vi "GetHighPrioritySensors.vi"   [LabVIEW 2020]
doc: "All high priority sensor reads and safety interlock calculations should be placed in this VI."
uses:
  <vilib>/Rock Robotics/WPI/DriverStation/WPI_DriverStationRobotMode2.ctl
  sensordata.vi
  robotoutputs.vi
  driverdata.vi
  refnumbers.vi
  GRNF_AI.vi
  GRNF_CTREMotor.vi
  <vilib>/Rock Robotics/WPI/ThirdParty/Phoenix-LabVIEW/Motor Controller/Get/CTRE_Phoenix_MotorController_GetSelectedSensorData.vi
  <vilib>/Rock Robotics/WPI/ThirdParty/Phoenix-LabVIEW/Motor Controller/Get/CTRE_Phoenix_MotorController_GetLimitSwitchStates.vi
  robotconstants.vi
types:
  T1 = typedef "WPI_DriverStationRobotMode2.ctl" = enum16{"Autonomous Disabled", "Autonomous Enabled", "Teleop Disabled", "Teleop Enabled", "Disconnected", "Finish", "Test Disabled", "Test Enabled", "Emergency Stopped"}
  T2 = enum16{"Low Gear", "High Gear", "Transiting", "Unknown", "Force Low Gear"}
  T3 = typedef "WPI_AnalogChannelDevRef.ctl" = cluster{"DevStatus":errorcluster, "Analog Channel":T4}
  T4 = typedef "FPGA_AIChannel.ctl" = enum8{"AI 0", "AI 1", "AI 2", "AI 3", "AI MXP 0", "AI MXP 1", "AI MXP 2", "AI MXP 3", "Invalid"}
  T5 = typedef "WPI_MotorControlDeviceRef.ctl" = cluster{"DeviceStatus":errorcluster, "Type":T6, "PWM":cluster{"PWM Channel":T7, "DeadBand":T8}, "CAN":cluster{"Device Number":u8, "SetOutput VI Ref":variant, "GetOutput VI Ref":variant, "Enable VI Ref":variant, "Disable VI Ref":variant, "Data":variant}, "Invert":bool, "DIO PWM":cluster{"PWM \"Enable\" Channel":T7, "DIOChannel":T9, "PWM Rate":dbl}}
  T6 = typedef "WPI_MotorControlType.ctl" = enum16{"PWM", "CAN", "DIO PWM"}
  T7 = typedef "FPGA_DIOPWMChannel.ctl" = enum8{"PWM 0", "PWM 1", "PWM 2", "PWM 3", "PWM 4", "PWM 5", "PWM 6", "PWM 7", "PWM 8", "PWM 9", "PWM MXP 0", "PWM MXP 1", "PWM MXP 2", "PWM MXP 3", "PWM MXP 4", "PWM MXP 5", "PWM MXP 6", "PWM MXP 7", "PWM MXP 8", "PWM MXP 9", "Invalid"}
  T8 = typedef "WPI_PWMDeadband.ctl" = cluster{"Name":string, "maxPositivePwm":i32, "minPositivePwm":i32, "centerPwm":i32, "maxNegativePwm":i32, "minNegativePwm":i32, "angularRange":u16}
  T9 = typedef "FPGA_DIOChannel.ctl" = enum8{"DIO 0", "DIO 1", "DIO 2", "DIO 3", "DIO 4", "DIO 5", "DIO 6", "DIO 7", "DIO 8", "DIO 9", "DIO MXP 0", "DIO MXP 1", "DIO MXP 2", "DIO MXP 3", "DIO MXP 4", "DIO MXP 5", "DIO MXP 6", "DIO MXP 7", "DIO MXP 8", "DIO MXP 9", "DIO MXP 10", "DIO MXP 11", "DIO MXP 12", "DIO MXP 13", "DIO MXP 14", "DIO MXP 15", "SPI Port CS1", "SPI Port CS2", "SPI Port CS3", "SPI Port MISO", "SPI Port MOSI", "Invalid"}
  T10 = typedef "Color Sensor V3 DevRef.ctl" = cluster{"I2CDevRef":T11}
  T11 = typedef "WPI_I2CDevRef.ctl" = cluster{"DevStatus":errorcluster, "Device Address":u8, "Handle":i32, "I2C Bus":T12}
  T12 = typedef "i2c_bus.ctl" = enum16{"I2C On-Board", "I2C MXP", "Invalid"}
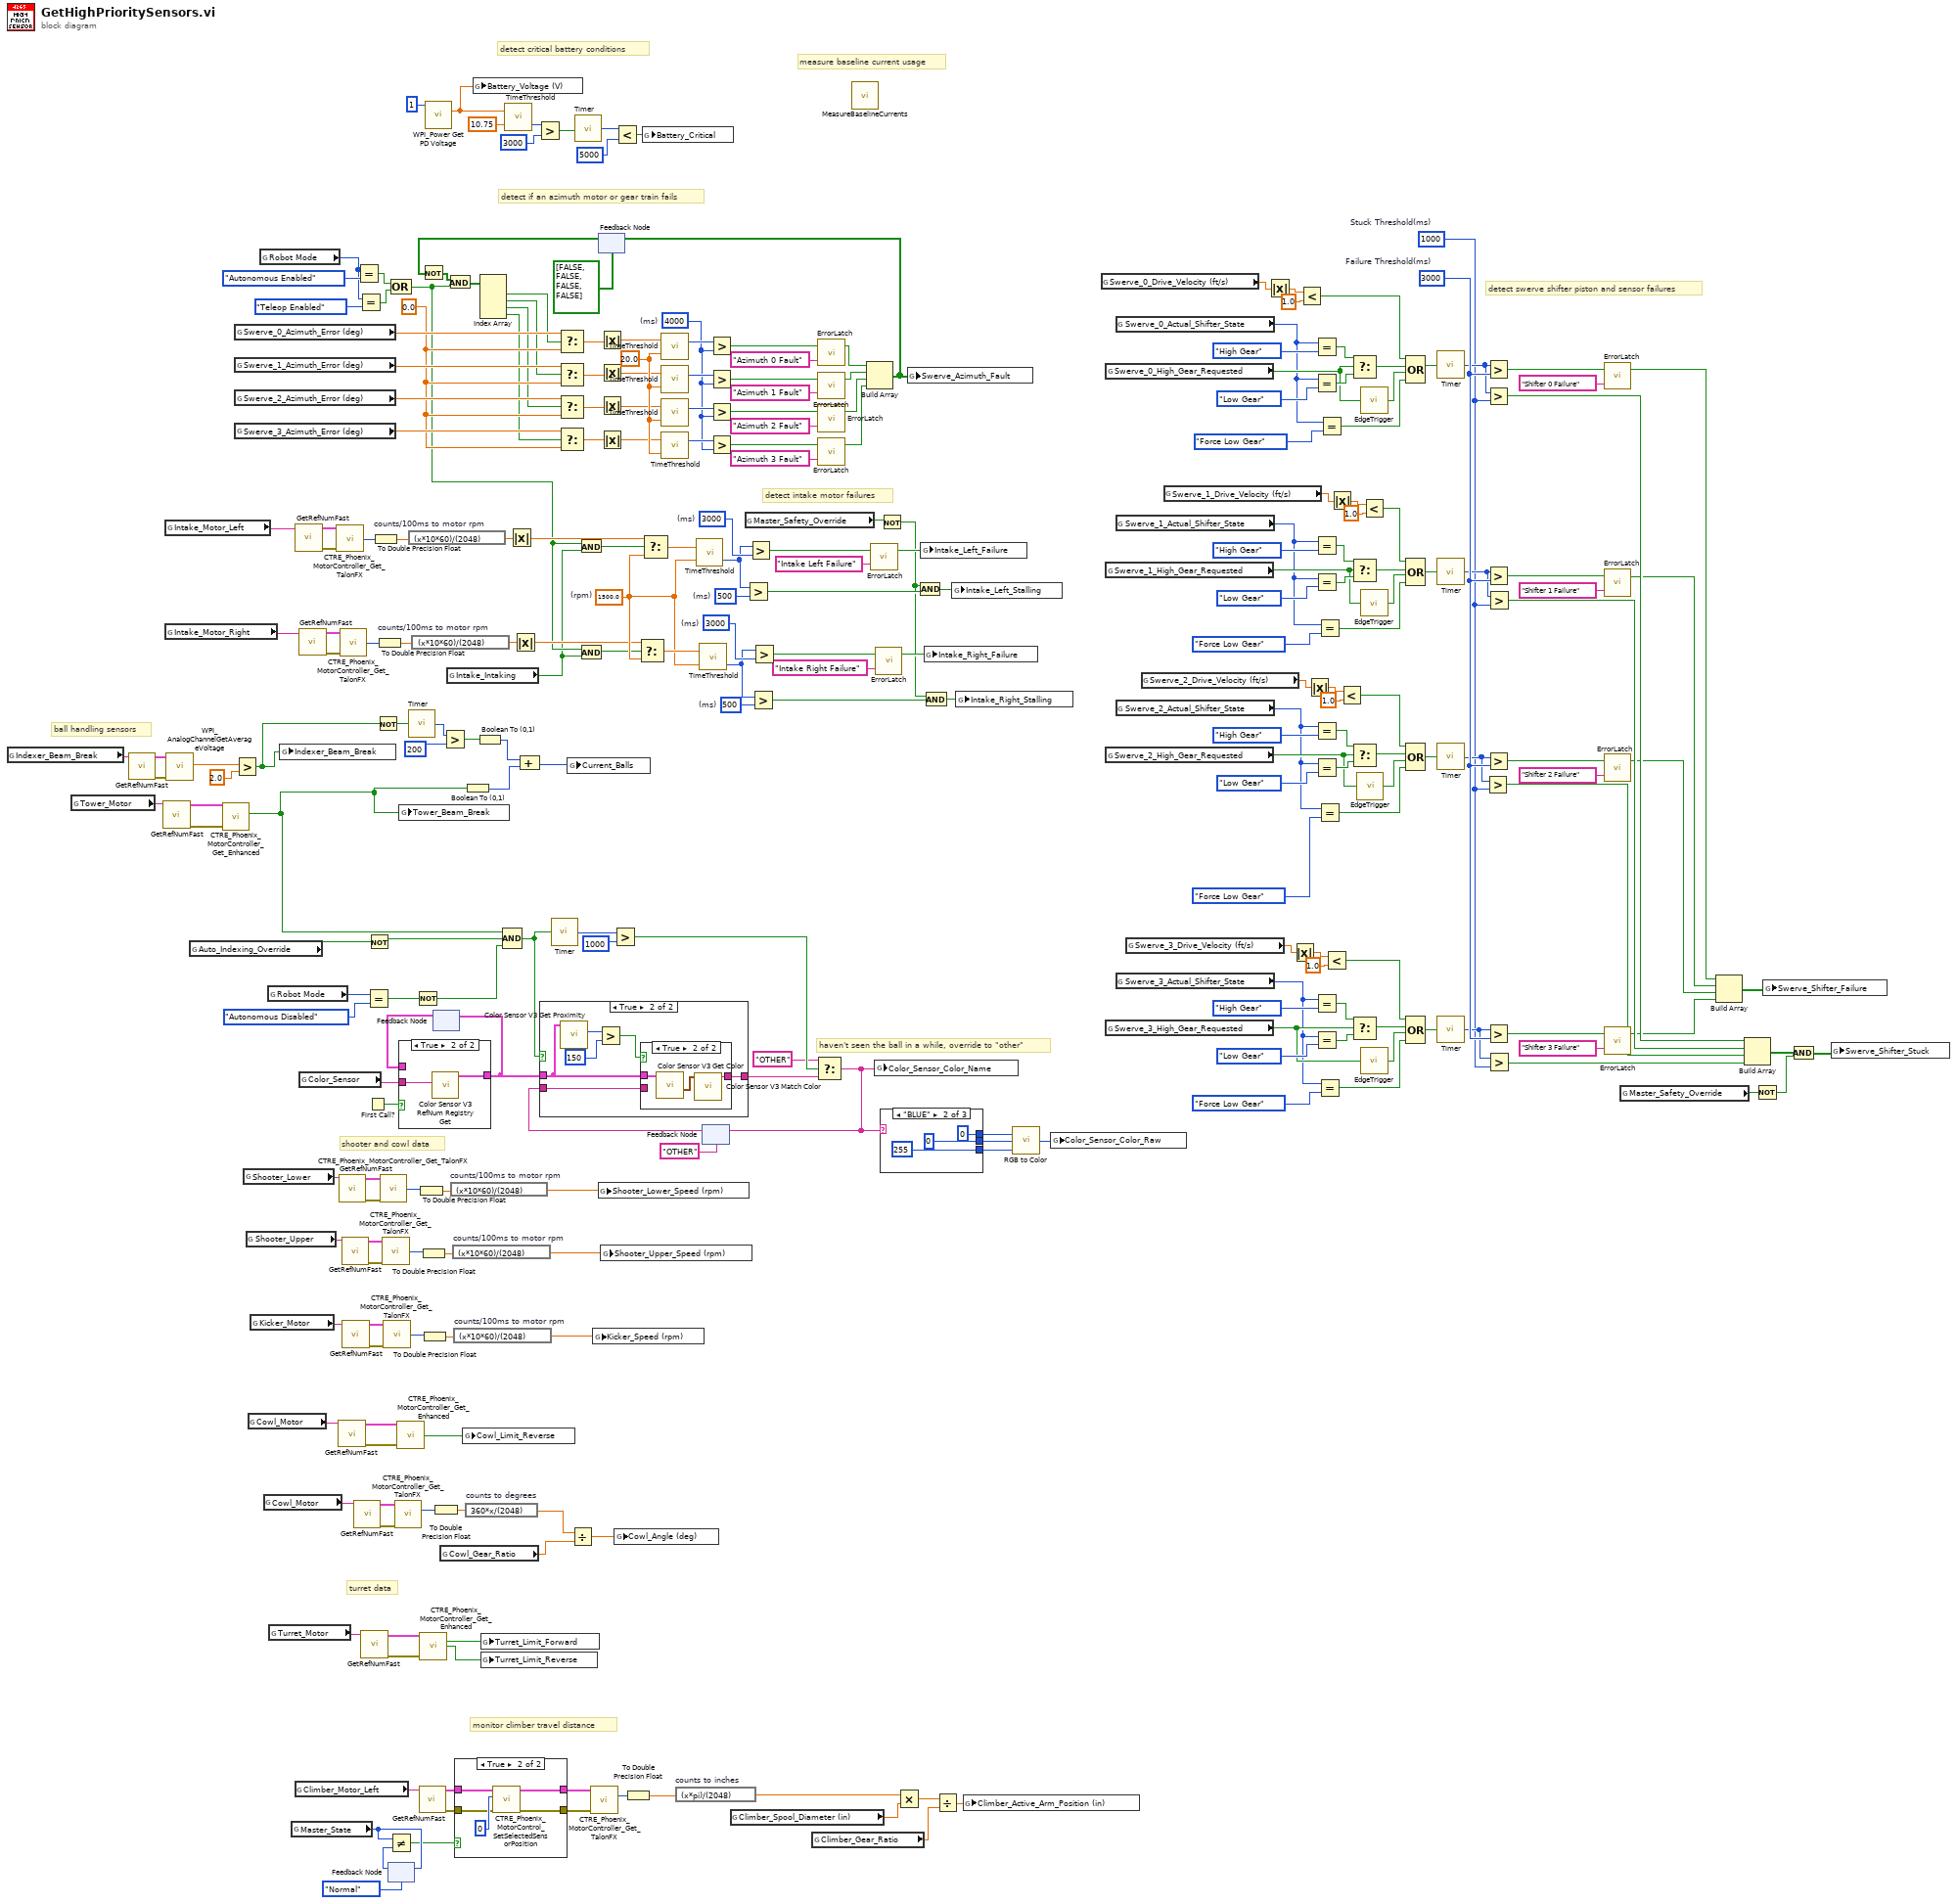
[diagram p0: block diagram]
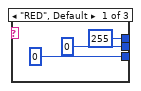
[diagram p5: hidden frame]
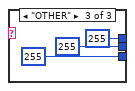
[diagram p6: hidden frame]
diagram:
  w22 = u32 500  # (ms)
  w24 = u32 500  # (ms)
  w129 = 1500.0  # (rpm)
  w136 = u32 3000  # (ms)
  w144 = u32 3000  # (ms)
  w198 = u32 1000  # Stuck Threshold(ms)
  w219 = u32 3000  # Failure Threshold(ms)
  w151 = 0.0
  w264 = u32 4000  # (ms)
  w263 = 20.0 ("Threshold")
  # "measure baseline current usage"
  # "monitor climber travel distance"
  # "haven't seen the ball in a while, override to \"other\""
  # "shooter and cowl data"
  # "turret data"
  # "detect intake motor failures"
  # "ball handling sensors"
  # "detect critical battery conditions"
  # "detect swerve shifter piston and sensor failures"
  # "detect if an azimuth motor or gear train fails"
  n1 = global read "refnumbers.vi" "Indexer_Beam_Break"() -> (w124:string)
  n2 = global read "refnumbers.vi" "Tower_Motor"() -> (w56:string)
  n3 = call-poly "GetRefNumFast.vi"("RefNum Name"=w124) -> ("Error"=w122:errorcluster, "Device Reference"=w123:T3)  [unwired: 5 in]
  n4 = call-poly "GetRefNumFast.vi"("RefNum Name"=w56) -> ("Error"=w54:errorcluster, "Device Reference"=w55:T5)  [unwired: 5 in]
  n5 = global read "refnumbers.vi" "Intake_Motor_Left"() -> (w149:string)
  n6 = global read "refnumbers.vi" "Intake_Motor_Right"() -> (w141:string)
  n7 = call <vilib>:"WPI_AnalogChannelGetAverageVoltage.vi"("error in (no error)"=w122, "AIDeviceRef"=w123) -> ("Voltage"=w150:dbl)  [unwired: 7 in, 2 out]
  n8 = global read "driverdata.vi" "Auto_Indexing_Override"() -> (w2:bool)
  n9 = call-poly <vilib>:"CTRE_Phoenix_MotorController_Get_Enhanced.vi"("PhoenixMotorControlDevRef"=w55, "error in"=w54) -> ("Forward Limit Closed?"=w3:bool)  [unwired: 10 in, 3 out]
  n10 = Greater?(x=w150, y=2.0) -> (0:w48:bool)
  n11 = global read "robotoutputs.vi" "Swerve_0_Azimuth_Error (deg)"() -> (w247:dbl)
  n12 = global read "robotoutputs.vi" "Swerve_1_Azimuth_Error (deg)"() -> (w246:dbl)
  n13 = global read "robotoutputs.vi" "Swerve_2_Azimuth_Error (deg)"() -> (w245:dbl)
  n14 = global read "robotoutputs.vi" "Swerve_3_Azimuth_Error (deg)"() -> (w244:dbl)
  n15 = global read "refnumbers.vi" "Shooter_Lower"() -> (w108:string)
  n16 = global read "refnumbers.vi" "Shooter_Upper"() -> (w102:string)
  n17 = global read "refnumbers.vi" "Cowl_Motor"() -> (w97:string)
  n18 = global read "refnumbers.vi" "Kicker_Motor"() -> (w7:string)
  n19 = global read "driverdata.vi" "Robot Mode"() -> (w256:T1)
  n20 = global read "refnumbers.vi" "Cowl_Motor"() -> (w94:string)
  n21 = global read "driverdata.vi" "Robot Mode"() -> (w79:T1)
  n22 = global read "refnumbers.vi" "Turret_Motor"() -> (w115:string)
  n23 = global write "sensordata.vi" "Indexer_Beam_Break"(w48) -> ()
  n24 = global read "robotoutputs.vi" "Master_State"() -> (w35:enum16{"Normal", "Climb"})
  n25 = global read "refnumbers.vi" "Climber_Motor_Left"() -> (w45:string)
  n26 = call-poly "GetRefNumFast.vi"("RefNum Name"=w149) -> ("Error"=w147:errorcluster, "Device Reference"=w148:T5)  [unwired: 5 in]
  n27 = call-poly "GetRefNumFast.vi"("RefNum Name"=w141) -> ("Error"=w139:errorcluster, "Device Reference"=w140:T5)  [unwired: 5 in]
  n28 = global read "refnumbers.vi" "Color_Sensor"() -> (w126:string)
  n29 = call-poly <vilib>:"CTRE_Phoenix_MotorController_Get_TalonFX.vi"("PhoenixMotorControlDevRef"=w148, "error in"=w147) -> ("Velocity (Raw Sensor Units per 100 ms)"=w146:i32)  [unwired: 10 in, 3 out]
  n30 = call-poly "GetRefNumFast.vi"("RefNum Name"=w97) -> ("Error"=w95:errorcluster, "Device Reference"=w96:T5)  [unwired: 5 in]
  n31 = call-poly "GetRefNumFast.vi"("RefNum Name"=w108) -> ("Error"=w106:errorcluster, "Device Reference"=w107:T5)  [unwired: 5 in]
  n32 = call-poly <vilib>:"CTRE_Phoenix_MotorController_Get_TalonFX.vi"("PhoenixMotorControlDevRef"=w140, "error in"=w139) -> ("Velocity (Raw Sensor Units per 100 ms)"=w138:i32)  [unwired: 10 in, 3 out]
  n33 = call-poly "GetRefNumFast.vi"("RefNum Name"=w102) -> ("Error"=w100:errorcluster, "Device Reference"=w101:T5)  [unwired: 5 in]
  n34 = call-poly "GetRefNumFast.vi"("RefNum Name"=w7) -> ("Error"=w5:errorcluster, "Device Reference"=w6:T5)  [unwired: 5 in]
  n35 = call-poly "GetRefNumFast.vi"("RefNum Name"=w94) -> ("Error"=w92:errorcluster, "Device Reference"=w93:T5)  [unwired: 5 in]
  n36 = Equal?(x=w256, y=WPI_DriverStationRobotMode2."Autonomous Enabled") -> (x = y?=w255:bool)
  n37 = Equal?(x=w256, y=WPI_DriverStationRobotMode2."Teleop Enabled") -> (x = y?=w254:bool)
  n38 = call-poly "GetRefNumFast.vi"("RefNum Name"=w115) -> ("Error"=w113:errorcluster, "Device Reference"=w114:T5)  [unwired: 5 in]
  n39 = Equal?(x=w79, y=WPI_DriverStationRobotMode2."Autonomous Disabled" ("Robot Mode")) -> (x = y?=w69:bool)
  n40 = First Call?() -> (First Call?: T/F=w127:bool)
  n41 = Not(x=w2) -> (.not. x?=w1:bool)
  n42 = To Double Precision Float(number=w146) -> (double precision float=w145:dbl)
  n43 = Not(x=w48) -> (.not. x?=w46:bool)
  n44 = To Double Precision Float(number=w138) -> (double precision float=w137:dbl)
  n45 = call-poly <vilib>:"CTRE_Phoenix_MotorController_Get_TalonFX.vi"("PhoenixMotorControlDevRef"=w107, "error in"=w106) -> ("Velocity (Raw Sensor Units per 100 ms)"=w109:i32)  [unwired: 10 in, 3 out]
  n46 = call-poly <vilib>:"CTRE_Phoenix_MotorController_Get_TalonFX.vi"("PhoenixMotorControlDevRef"=w101, "error in"=w100) -> ("Velocity (Raw Sensor Units per 100 ms)"=w103:i32)  [unwired: 10 in, 3 out]
  n47 = call-poly <vilib>:"CTRE_Phoenix_MotorController_Get_TalonFX.vi"("PhoenixMotorControlDevRef"=w6, "error in"=w5) -> ("Velocity (Raw Sensor Units per 100 ms)"=w8:i32)  [unwired: 10 in, 3 out]
  n48 = feedback #1(enum16{"Normal", "Climb"}."Normal" ("Master_State")) -> (w36:enum16{"Normal", "Climb"})
  n49 = Not Equal?(x=w35, y=w36) -> (x != y?=w34:bool)
  n50 = feedback-in #1(w35) -> ()
  n51 = Compound Arithmetic op=OR(w255, w254) -> (w25:bool)
  n52 = call-poly <vilib>:"CTRE_Phoenix_MotorController_Get_TalonFX.vi"("PhoenixMotorControlDevRef"=w93, "error in"=w92) -> ("Position (Raw Sensor Units)"=w91:i32)  [unwired: 10 in, 3 out]
  n53 = call-poly <vilib>:"CTRE_Phoenix_MotorController_Get_Enhanced.vi"("PhoenixMotorControlDevRef"=w96, "error in"=w95) -> ("Reverse Limit Closed?"=w98:bool)  [unwired: 10 in, 3 out]
  n54 = global write "sensordata.vi" "Tower_Beam_Break"(w3) -> ()
  n55 = expression code="(x*10*60)/(2048)" "counts/100ms to motor rpm"(w145) -> (w128:dbl)
  n56 = call "Timer.vi"("Reset Timer"=w46) -> ("Time (ms)"=w53:u32)
  n57 = expression code="(x*10*60)/(2048)" "counts/100ms to motor rpm"(w137) -> (w133:dbl)
  n58 = Not(x=w69) -> (.not. x?=w29:bool)
  n59 = To Double Precision Float(number=w109) -> (double precision float=w110:dbl)
  n60 = call-poly "GetRefNumFast.vi"("RefNum Name"=w45) -> ("Error"=w39:errorcluster, "Device Reference"=w40:T5)  [unwired: 5 in]
  n61 = call-poly <vilib>:"CTRE_Phoenix_MotorController_Get_Enhanced.vi"("PhoenixMotorControlDevRef"=w114, "error in"=w113) -> ("Forward Limit Closed?"=w112:bool, "Reverse Limit Closed?"=w111:bool)  [unwired: 10 in, 2 out]
  n62 = To Double Precision Float(number=w103) -> (double precision float=w104:dbl)
  n63 = To Double Precision Float(number=w8) -> (double precision float=w9:dbl)
  n64 = call <vilib>:"WPI_Power Get PD Voltage.vi"("Power Distribution Panel (def)"=u8 1) -> ("voltage (V)"=w153:dbl)  [unwired: 13 in, 1 out]
  n65 = feedback #2() -> (w125:T10)  [unwired: 1 in]
  n66 = case shown="True" w127 {
    tunnel: [w272 w273] -> w68
    tunnel: w125 -> [w272 _]
    tunnel: w126 -> [_ w274]
    frame False {
    }
    frame True {
      n67 = call <vilib>:"Color Sensor V3 RefNum Registry Get.vi"("refnum name"=w274) -> ("ColorSensorDevRef"=w273:T10)  [unwired: 9 in, 1 out]
    }
  }
  n68 = feedback-in #2(w68) -> ()
  n69 = To Double Precision Float(number=w91) -> (double precision float=w90:dbl)
  n70 = global read "robotconstants.vi" "Cowl_Gear_Ratio"() -> (w88:dbl)
  n71 = Greater?(x=w53, y=u32 200) -> (0:w52:bool)
  n72 = global read "robotoutputs.vi" "Intake_Intaking"() -> (w20:bool)
  n73 = expression code="(x*10*60)/(2048)" "counts/100ms to motor rpm"(w110) -> (w105:dbl)
  n74 = expression code="(x*10*60)/(2048)" "counts/100ms to motor rpm"(w104) -> (w99:dbl)
  n75 = expression code="(x*10*60)/(2048)" "counts/100ms to motor rpm"(w9) -> (w4:dbl)
  n76 = case shown="True" w34 {
    tunnel: w40 -> [w276 w280]
    tunnel: w39 -> [w275 w279]
    tunnel: [w276 w278] -> w37
    tunnel: [w275 w277] -> w38
    frame False {
    }
    frame True {
      n77 = call <vilib>:"CTRE_Phoenix_MotorControl_SetSelectedSensorPosition.vi"("error in (no error)"=w279, "New Sensor Position"=0, "PhoenixMotorControlDevRef"=w280) -> ("error out"=w277:errorcluster, "PhoenixMotorControlDevRef"=w278:T5)  [unwired: 7 in]
    }
  }
  n78 = global write "sensordata.vi" "Cowl_Limit_Reverse"(w98) -> ()
  n79 = Boolean To (0,1)(Boolean=w3) -> (0, 1=w50:i16)
  n80 = expression code="360*x/(2048)" "counts to degrees"(w90) -> (w89:dbl)
  n81 = global write "sensordata.vi" "Battery_Voltage (V)"(w153) -> ()
  n82 = Boolean To (0,1)(Boolean=w52) -> (0, 1=w51:i16)
  n83 = global write "sensordata.vi" "Turret_Limit_Forward"(w112) -> ()
  n84 = global write "sensordata.vi" "Turret_Limit_Reverse"(w111) -> ()
  n85 = Compound Arithmetic op=AND(w3, w1, w29) -> (w67:bool)
  n86 = call "TimeThreshold.vi"("Threshold"=10.75, "Current Value"=w153) -> ("Time Below Threshold (ms)"=w270:u32)  [unwired: 1 out]
  n87 = Absolute Value(x=w128) -> (abs(x)=w28:dbl)
  n88 = Absolute Value(x=w133) -> (abs(x)=w27:dbl)
  n89 = Compound Arithmetic op=ADD(w51, w50) -> (w49:i16)
  n90 = Greater?(x=w270, y=u32 3000) -> (0:w13:bool)
  n91 = call "Timer.vi"("Reset Timer"=w67) -> ("Time (ms)"=w86:u32)
  n92 = global write "sensordata.vi" "Current_Balls"(w49) -> ()
  n93 = Divide(x=w89, y=w88) -> (x/y=w87:dbl)
  n94 = call "Timer.vi"("Reset Timer"=w13) -> ("Time (ms)"=w12:u32)
  n95 = And(x=w25, y=w20) -> (x .and. y?=w130:bool)
  n96 = And(x=w25, y=w20) -> (x .and. y?=w26:bool)
  n97 = call-poly <vilib>:"CTRE_Phoenix_MotorController_Get_TalonFX.vi"("PhoenixMotorControlDevRef"=w37, "error in"=w38) -> ("Position (Raw Sensor Units)"=w43:i32)  [unwired: 10 in, 3 out]
  n98 = global write "sensordata.vi" "Kicker_Speed (rpm)"(w4) -> ()
  n99 = feedback #3(bool[] [FALSE, FALSE, FALSE, FALSE]) -> (w77:bool[])
  n100 = Not(x=w77) -> (.not. x?=w76:bool[])
  n101 = And(x=w76, y=w25) -> (x .and. y?=w75:bool[])
  n102 = Index Array(array=w75) -> (element #1=w71:bool, element #2=w72:bool, element #3=w73:bool, element #4=w74:bool)  [unwired: 4 in]
  n103 = Select(t=w247, s=w71, f=w151) -> (s? t:f=w243:dbl)
  n104 = Select(t=w246, s=w72, f=w151) -> (s? t:f=w242:dbl)
  n105 = Select(t=w245, s=w73, f=w151) -> (s? t:f=w241:dbl)
  n106 = Select(t=w244, s=w74, f=w151) -> (s? t:f=w240:dbl)
  n107 = global write "sensordata.vi" "Shooter_Lower_Speed (rpm)"(w105) -> ()
  n108 = Absolute Value(x=w243) -> (abs(x)=w262:dbl)
  n109 = Absolute Value(x=w242) -> (abs(x)=w261:dbl)
  n110 = Absolute Value(x=w241) -> (abs(x)=w260:dbl)
  n111 = Absolute Value(x=w240) -> (abs(x)=w259:dbl)
  n112 = global write "sensordata.vi" "Shooter_Upper_Speed (rpm)"(w99) -> ()
  n113 = Greater?(x=w86, y=u32 1000) -> (0:w84:bool)
  n114 = Less?(x=w12, y=u32 5000) -> (x < y?=w11:bool)
  n115 = global write "sensordata.vi" "Cowl_Angle (deg)"(w87) -> ()
  n116 = To Double Precision Float(number=w43) -> (double precision float=w44:dbl)
  n117 = Select(t=w27, s=w26, f=w129) -> (s? t:f=w131:dbl)
  n118 = global write "sensordata.vi" "Battery_Critical"(w11) -> ()
  n119 = Select(t=w28, s=w130, f=w129) -> (s? t:f=w132:dbl)
  n120 = call "TimeThreshold.vi"("Threshold"=w263, "Current Value"=w262) -> ("Time Above Threshold (ms)"=w268:u32)  [unwired: 1 out]
  n121 = call "TimeThreshold.vi"("Threshold"=w263, "Current Value"=w261) -> ("Time Above Threshold (ms)"=w267:u32)  [unwired: 1 out]
  n122 = call "TimeThreshold.vi"("Threshold"=w263, "Current Value"=w260) -> ("Time Above Threshold (ms)"=w266:u32)  [unwired: 1 out]
  n123 = call "TimeThreshold.vi"("Threshold"=w263, "Current Value"=w259) -> ("Time Above Threshold (ms)"=w265:u32)  [unwired: 1 out]
  n124 = expression code="(x*pi)/(2048)" "counts to inches"(w44) -> (w32:dbl)
  n125 = call "TimeThreshold.vi"("Threshold"=w129, "Current Value"=w132) -> ("Time Below Threshold (ms)"=w23:u32)  [unwired: 1 out]
  n126 = call "TimeThreshold.vi"("Threshold"=w129, "Current Value"=w131) -> ("Time Below Threshold (ms)"=w21:u32)  [unwired: 1 out]
  n127 = feedback #4("OTHER" ("Matched Color Name")) -> (w116:string)
  n128 = case shown="True" w67 {
    tunnel: w68 -> [_ w287]
    tunnel: [w282 w288] -> w81
    tunnel: w116 -> [w282 w286]
    frame False {
    }
    frame True {
      n129 = call <vilib>:"Color Sensor V3 Get Proximity.vi"("ColorSensorDevRef"=w287) -> ("Proximity"=w285:u16)  [unwired: 8 in, 2 out]
      n130 = Greater?(x=w285, y=u16 150) -> (0:w283:bool)
      n131 = case shown="True" w283 {
        tunnel: [w289 w291] -> w288
        tunnel: w287 -> [_ w290]
        tunnel: w286 -> [w289 _]
        frame False {
        }
        frame True {
          n132 = call <vilib>:"Color Sensor V3 Get Color.vi"("ColorSensorDevRef"=w290) -> ("Normalized Color"=w292:cluster{"R":dbl, "G":dbl, "B":dbl})  [unwired: 7 in, 3 out]
          n133 = call <vilib>:"Color Sensor V3 Match Color.vi"("Measured Color"=w292) -> ("Matched Color Name"=w291:string)  [unwired: 8 in, 2 out]
        }
      }
    }
  }
  n134 = Greater?(x=w268, y=w264) -> (0:w250:bool)
  n135 = Greater?(x=w267, y=w264) -> (0:w249:bool)
  n136 = Greater?(x=w266, y=w264) -> (0:w155:bool)
  n137 = Greater?(x=w265, y=w264) -> (0:w248:bool)
  n138 = global read "robotconstants.vi" "Climber_Spool_Diameter (in)"() -> (w30:dbl)
  n139 = global read "driverdata.vi" "Master_Safety_Override"() -> (w19:bool)
  n140 = Greater?(x=w23, y=w24) -> (0:w17:bool)
  n141 = Greater?(x=w23, y=w144) -> (0:w143:bool)
  n142 = Greater?(x=w21, y=w22) -> (0:w15:bool)
  n143 = Greater?(x=w21, y=w136) -> (0:w135:bool)
  n144 = global read "robotconstants.vi" "Climber_Gear_Ratio"() -> (w42:dbl)
  n145 = Select(t="OTHER" ("Matched Color Name"), s=w84, f=w81) -> (s? t:f=w82:string)
  n146 = feedback-in #4(w82) -> ()
  n147 = call "ErrorLatch.vi"("Error Message"="Azimuth 0 Fault", "Trigger"=w250) -> ("Latched"=w176:bool)  [unwired: 1 in]
  n148 = call "ErrorLatch.vi"("Error Message"="Azimuth 1 Fault", "Trigger"=w249) -> ("Latched"=w253:bool)  [unwired: 1 in]
  n149 = call "ErrorLatch.vi"("Error Message"="Azimuth 2 Fault", "Trigger"=w155) -> ("Latched"=w252:bool)  [unwired: 1 in]
  n150 = call "ErrorLatch.vi"("Error Message"="Azimuth 3 Fault", "Trigger"=w248) -> ("Latched"=w251:bool)  [unwired: 1 in]
  n151 = call "MeasureBaselineCurrents.vi"() -> ()  [unwired: 12 in]
  n152 = Build Array(w176, w253, w252, w251) -> (w78:bool[])
  n153 = feedback-in #3(w78) -> ()
  n154 = call "ErrorLatch.vi"("Error Message"="Intake Left Failure", "Trigger"=w143) -> ("Latched"=w142:bool)  [unwired: 1 in]
  n155 = global write "sensordata.vi" "Color_Sensor_Color_Name"(w82) -> ()
  n156 = call "ErrorLatch.vi"("Error Message"="Intake Right Failure", "Trigger"=w135) -> ("Latched"=w134:bool)  [unwired: 1 in]
  n157 = Not(x=w19) -> (.not. x?=w16:bool)
  n158 = case shown="\"BLUE\"" w82 {
    tunnel: [u8 255 ("R") u8 0 ("R") u8 255 ("R")] -> w120
    tunnel: [u8 0 ("R") u8 0 ("R") u8 255 ("R")] -> w119
    tunnel: [u8 0 ("R") u8 255 ("R") u8 255 ("R")] -> w118
    frame "RED", Default {
    }
    frame "BLUE" {
    }
    frame "OTHER" {
    }
  }
  n159 = Multiply(x=w32, y=w30) -> (x*y=w31:dbl)
  n160 = global write "sensordata.vi" "Swerve_Azimuth_Fault"(w78) -> ()
  n161 = And(x=w16, y=w17) -> (x .and. y?=w18:bool)
  n162 = global write "sensordata.vi" "Intake_Left_Failure"(w142) -> ()
  n163 = And(x=w16, y=w15) -> (x .and. y?=w14:bool)
  n164 = global write "sensordata.vi" "Intake_Right_Failure"(w134) -> ()
  n165 = Divide(x=w31, y=w42) -> (x/y=w41:dbl)
  n166 = global write "sensordata.vi" "Intake_Left_Stalling"(w18) -> ()
  n167 = global write "sensordata.vi" "Intake_Right_Stalling"(w14) -> ()
  n168 = global write "sensordata.vi" "Climber_Active_Arm_Position (in)"(w41) -> ()
  n169 = call <vilib>:"RGB to Color.vi"("B"=w118, "G"=w119, "R"=w120) -> ("Color"=w121:u32)
  n170 = global write "sensordata.vi" "Color_Sensor_Color_Raw"(w121) -> ()
  n171 = global read "sensordata.vi" "Swerve_0_Drive_Velocity (ft/s)"() -> (w193:dbl)
  n172 = global read "robotoutputs.vi" "Swerve_0_High_Gear_Requested"() -> (w218:bool)
  n173 = global read "robotoutputs.vi" "Swerve_1_High_Gear_Requested"() -> (w211:bool)
  n174 = global read "robotoutputs.vi" "Swerve_2_High_Gear_Requested"() -> (w208:bool)
  n175 = global read "robotoutputs.vi" "Swerve_3_High_Gear_Requested"() -> (w203:bool)
  n176 = global read "sensordata.vi" "Swerve_0_Actual_Shifter_State"() -> (w165:T2)
  n177 = global read "sensordata.vi" "Swerve_1_Actual_Shifter_State"() -> (w168:T2)
  n178 = global read "sensordata.vi" "Swerve_2_Actual_Shifter_State"() -> (w171:T2)
  n179 = global read "sensordata.vi" "Swerve_3_Actual_Shifter_State"() -> (w174:T2)
  n180 = global read "sensordata.vi" "Swerve_3_Drive_Velocity (ft/s)"() -> (w181:dbl)
  n181 = global read "sensordata.vi" "Swerve_2_Drive_Velocity (ft/s)"() -> (w185:dbl)
  n182 = global read "sensordata.vi" "Swerve_1_Drive_Velocity (ft/s)"() -> (w189:dbl)
  n183 = Absolute Value(x=w193) -> (abs(x)=w192:dbl)
  n184 = Absolute Value(x=w181) -> (abs(x)=w180:dbl)
  n185 = Less?(x=w192, y=1.0) -> (x < y?=w190:bool)
  n186 = Absolute Value(x=w185) -> (abs(x)=w184:dbl)
  n187 = Equal?(x=w165, y=T2."High Gear") -> (x = y?=w238:bool)
  n188 = Equal?(x=w165, y=T2."Low Gear") -> (x = y?=w236:bool)
  n189 = Equal?(x=w168, y=T2."High Gear") -> (x = y?=w233:bool)
  n190 = Equal?(x=w168, y=T2."Low Gear") -> (x = y?=w231:bool)
  n191 = Equal?(x=w171, y=T2."High Gear") -> (x = y?=w228:bool)
  n192 = Equal?(x=w171, y=T2."Low Gear") -> (x = y?=w226:bool)
  n193 = Equal?(x=w174, y=T2."High Gear") -> (x = y?=w223:bool)
  n194 = Equal?(x=w174, y=T2."Low Gear") -> (x = y?=w221:bool)
  n195 = Equal?(x=w168, y=T2."Force Low Gear") -> (x = y?=w167:bool)
  n196 = Equal?(x=w171, y=T2."Force Low Gear") -> (x = y?=w170:bool)
  n197 = Equal?(x=w174, y=T2."Force Low Gear") -> (x = y?=w173:bool)
  n198 = Equal?(x=w165, y=T2."Force Low Gear") -> (x = y?=w164:bool)
  n199 = Less?(x=w180, y=1.0) -> (x < y?=w178:bool)
  n200 = Absolute Value(x=w189) -> (abs(x)=w188:dbl)
  n201 = Less?(x=w184, y=1.0) -> (x < y?=w182:bool)
  n202 = Select(t=w238, s=w218, f=w236) -> (s? t:f=w216:bool)
  n203 = Select(t=w233, s=w211, f=w231) -> (s? t:f=w213:bool)
  n204 = Select(t=w228, s=w208, f=w226) -> (s? t:f=w210:bool)
  n205 = Select(t=w223, s=w203, f=w221) -> (s? t:f=w206:bool)
  n206 = call "EdgeTrigger.vi"("Input Signal"=w208) -> ("All Edge Trigger"=w209:bool)  [unwired: 2 out]
  n207 = call "EdgeTrigger.vi"("Input Signal"=w218) -> ("All Edge Trigger"=w217:bool)  [unwired: 2 out]
  n208 = Less?(x=w188, y=1.0) -> (x < y?=w186:bool)
  n209 = call "EdgeTrigger.vi"("Input Signal"=w211) -> ("All Edge Trigger"=w214:bool)  [unwired: 2 out]
  n210 = call "EdgeTrigger.vi"("Input Signal"=w203) -> ("All Edge Trigger"=w204:bool)  [unwired: 2 out]
  n211 = Compound Arithmetic op=OR(w190, w216, w217, w164) -> (w215:bool)
  n212 = Compound Arithmetic op=OR(w186, w213, w214, w167) -> (w212:bool)
  n213 = Compound Arithmetic op=OR(w182, w210, w209, w170) -> (w207:bool)
  n214 = Compound Arithmetic op=OR(w178, w206, w204, w173) -> (w205:bool)
  n215 = call "Timer.vi"("Reset Timer"=w215) -> ("Time (ms)"=w202:u32)
  n216 = call "Timer.vi"("Reset Timer"=w212) -> ("Time (ms)"=w201:u32)
  n217 = call "Timer.vi"("Reset Timer"=w207) -> ("Time (ms)"=w200:u32)
  n218 = call "Timer.vi"("Reset Timer"=w205) -> ("Time (ms)"=w199:u32)
  n219 = Greater?(x=w200, y=w198) -> (0:w158:bool)
  n220 = Greater?(x=w202, y=w219) -> (0:w235:bool)
  n221 = Greater?(x=w202, y=w198) -> (0:w162:bool)
  n222 = Greater?(x=w201, y=w219) -> (0:w230:bool)
  n223 = Greater?(x=w200, y=w219) -> (0:w225:bool)
  n224 = Greater?(x=w199, y=w219) -> (0:w220:bool)
  n225 = Greater?(x=w201, y=w198) -> (0:w160:bool)
  n226 = Greater?(x=w199, y=w198) -> (0:w157:bool)
  n227 = call "ErrorLatch.vi"("Error Message"="Shifter 0 Failure", "Trigger"=w235) -> ("Latched"=w163:bool)  [unwired: 1 in]
  n228 = call "ErrorLatch.vi"("Error Message"="Shifter 1 Failure", "Trigger"=w230) -> ("Latched"=w161:bool)  [unwired: 1 in]
  n229 = call "ErrorLatch.vi"("Error Message"="Shifter 2 Failure", "Trigger"=w225) -> ("Latched"=w159:bool)  [unwired: 1 in]
  n230 = call "ErrorLatch.vi"("Error Message"="Shifter 3 Failure", "Trigger"=w220) -> ("Latched"=w156:bool)  [unwired: 1 in]
  n231 = global read "driverdata.vi" "Master_Safety_Override"() -> (w197:bool)
  n232 = Build Array(w163, w161, w159, w156) -> (w177:bool[])
  n233 = Build Array(w162, w160, w158, w157) -> (w196:bool[])
  n234 = Not(x=w197) -> (.not. x?=w195:bool)
  n235 = global write "sensordata.vi" "Swerve_Shifter_Failure"(w177) -> ()
  n236 = And(x=w196, y=w195) -> (x .and. y?=w194:bool[])
  n237 = global write "sensordata.vi" "Swerve_Shifter_Stuck"(w194) -> ()
